vi "_Simple Demo.vi"() -> ()   [LabVIEW 2017]
panel:
  out "FPS":dbl(graph)
  out "new picture":picture
  in  "stop":bool
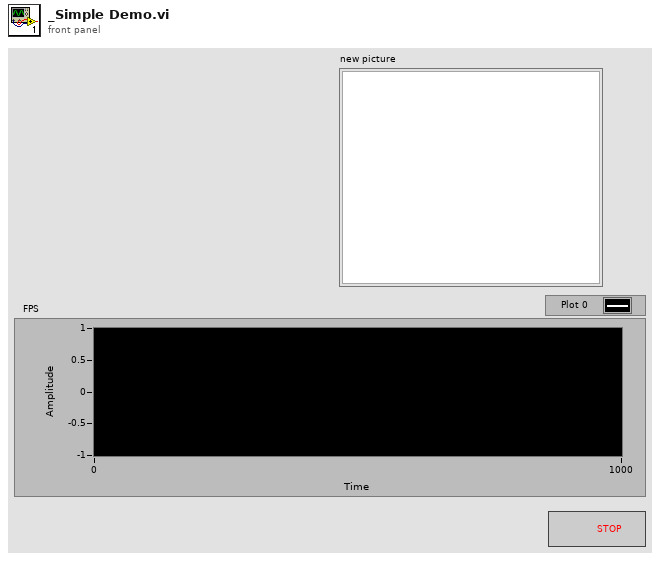
[diagram p1: front panel]
types:
  T1 = typedef "imagedata.ctl" = cluster{"image type":i32, "image depth":i32, "image":u8[], "mask":u8[], "colors":u32[], "Rectangle":cluster{"left":i16, "top":i16, "right":i16, "bottom":i16}}
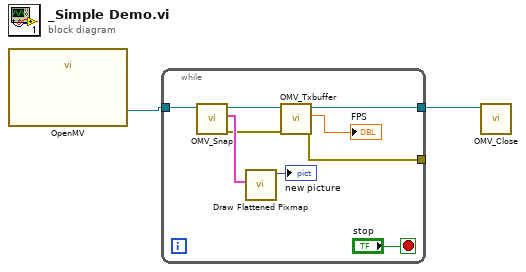
[diagram p0: block diagram]
diagram:
  n1 = call "OpenMV"() -> ("USB Connection out"=w1:refnum<visa-resource-name>)  [unwired: 11 in]
  n2 = while {
    tunnel: w1 -> [w11]
    tunnel: [w9] -> w2
    tunnel: [w3] -> _
    stop <- "stop" stop-if-true
    n3 = call "OMV_Snap.vi"("VISA Refnum in"=w11) -> ("error out"=w4:errorcluster, "image data"=w7:T1, "VISA Refnum out"=w10:refnum<visa-resource-name>)  [unwired: 8 in]
    n4 = call <vilib>:"Draw Flattened Pixmap.vi"("image data"=w7) -> ("new picture"=→"new picture":picture)  [unwired: 8 in]
    n5 = call "OMV_Txbuffer.vi"("error in (no error)"=w4, "VISA Refnum in"=w10) -> ("error out"=w3:errorcluster, "Data"=→"FPS":dbl, "VISA Refnum out"=w9:refnum<visa-resource-name>)  [unwired: 7 in]
  }
  n6 = call "OMV_Close.vi"("VISA Refnum in"=w2) -> ()  [unwired: 11 in]
